vi "TCP-KO-Send Command Receive I16.vi"(0 "connection ID":refnum<k5>, 7 "Command":string, 9 "timeout (ms)":i32=5000, 11 "error in (no error)":errorcluster) -> (4 "connection ID out":refnum<k5>, 6 "value":i16, 10 "result":i32, 15 "error out":errorcluster)   [LabVIEW 2020]
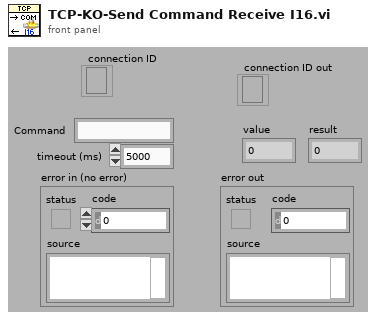
[diagram p1: front panel]
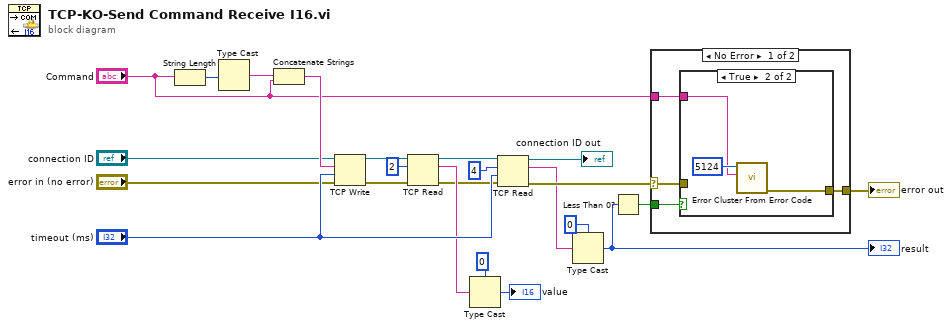
[diagram p0: block diagram]
diagram:
  n1 = String Length(string="Command") -> (length=w22:i32)
  n2 = Type Cast(x=w22) -> (*(type *) &x=w21:string)  [unwired: 1 in]
  n3 = Concatenate Strings(w21, "Command") -> (w23:string)
  n4 = TCP Write(connection ID="connection ID", data in=w23, error in (no error)="error in (no error)", 9:"timeout (ms)") -> (connection ID out=w11:refnum<k5>, error out=w10:errorcluster)  [unwired: 1 out]
  n5 = TCP Read(connection ID=w11, bytes to read=2, error in (no error)=w10) -> (connection ID out=w9:refnum<k5>, data out=w8:string, error out=w7:errorcluster)  [unwired: 2 in]
  n6 = Type Cast(type=i16 0, x=w8) -> (*(type *) &x=→"value":i16)
  n7 = TCP Read(connection ID=w9, bytes to read=4, error in (no error)=w7, 9:"timeout (ms)") -> (connection ID out=→"connection ID out":refnum<k5>, data out=w17:string, error out=w18:errorcluster)  [unwired: 1 in]
  n8 = Type Cast(type=0, x=w17) -> (*(type *) &x=w15:i32)
  "result" <- w15
  n9 = Less Than 0?(x=w15) -> (x < 0?=w14:bool)
  n10 = case shown="No Error" w18 {
    selector: w18 -> [w27 w32]
    tunnel: w14 -> [w26 _]
    tunnel: [w25 w32] -> w13
    tunnel: "Command" -> [w24 _]
    frame No Error {
      n11 = case shown="True" w26 {
        tunnel: [w28 w29] -> w25
        tunnel: w27 -> [w28 _]
        tunnel: w24 -> [_ w30]
        frame False {
        }
        frame True {
          n12 = call <vilib>:"Error Cluster From Error Code.vi"("error message (\"\")"=w30, "error code (0)"=5124) -> ("error out"=w29:errorcluster)  [unwired: 7 in]
        }
      }
    }
    frame Error {
    }
  }
  "error out" <- w13
